vi "filename-manage.vi"(6 "filename pattern":T2, 7 "filename-action":T1=enum."parse", 9 "folder":path=path "C:/data/Ultrasound/birdcage/Hg1201/Test", 11 "file name":string="f027_lsco2_122317.dat") -> (3 "filename OUT":string)   [LabVIEW 2018]
uses:
  filename-pattern.ctl
  filename-action.ctl
  <vilib>/Utility/libraryn.llb/Check if File or Folder Exists.vi
  <vilib>/regexp/Match Regular Expression.xnode
panel:
  out "unique index out":i32
  out "pattern 2":string="^(\\s+)(\\d+)_(.*)_(\\d\\d\\d\\d\\d\\d)\\.dat$"
  out "pattern":string="^(\\s+)(\\d+)_(.*)_(\\d\\d\\d\\d\\d\\d)\\.dat$"
  out "whole match":string
  out "offset past match":i32=-1
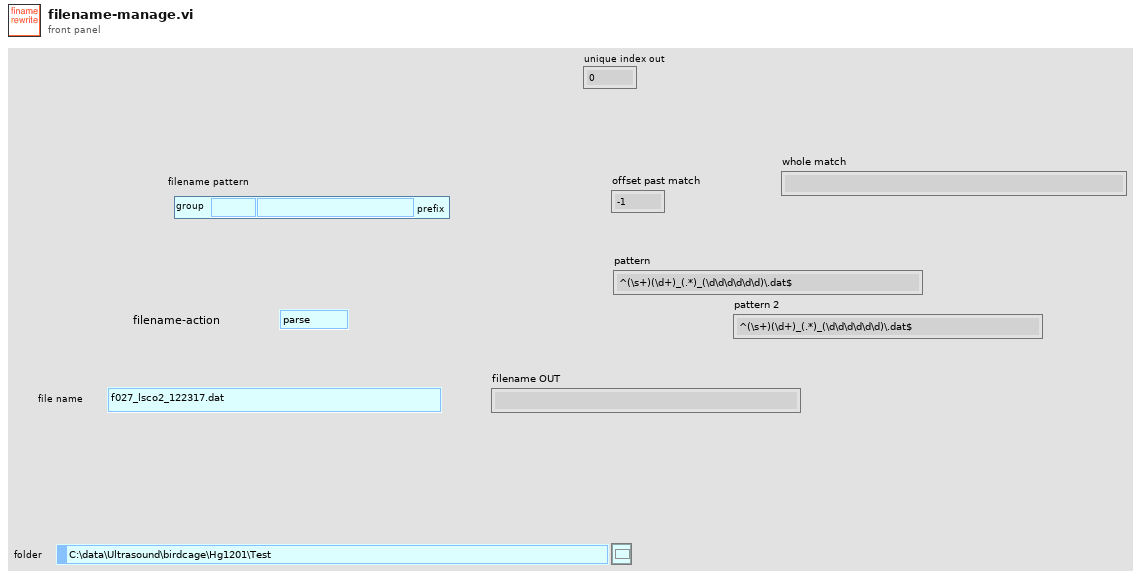
[diagram p1: front panel]
types:
  T1 = typedef "filename-action.ctl" = enum16{"rewrite", "parse", "force pattern", "uniquenum"}
  T2 = typedef "filename-pattern.ctl" = cluster{"prefix":string, "group":string}
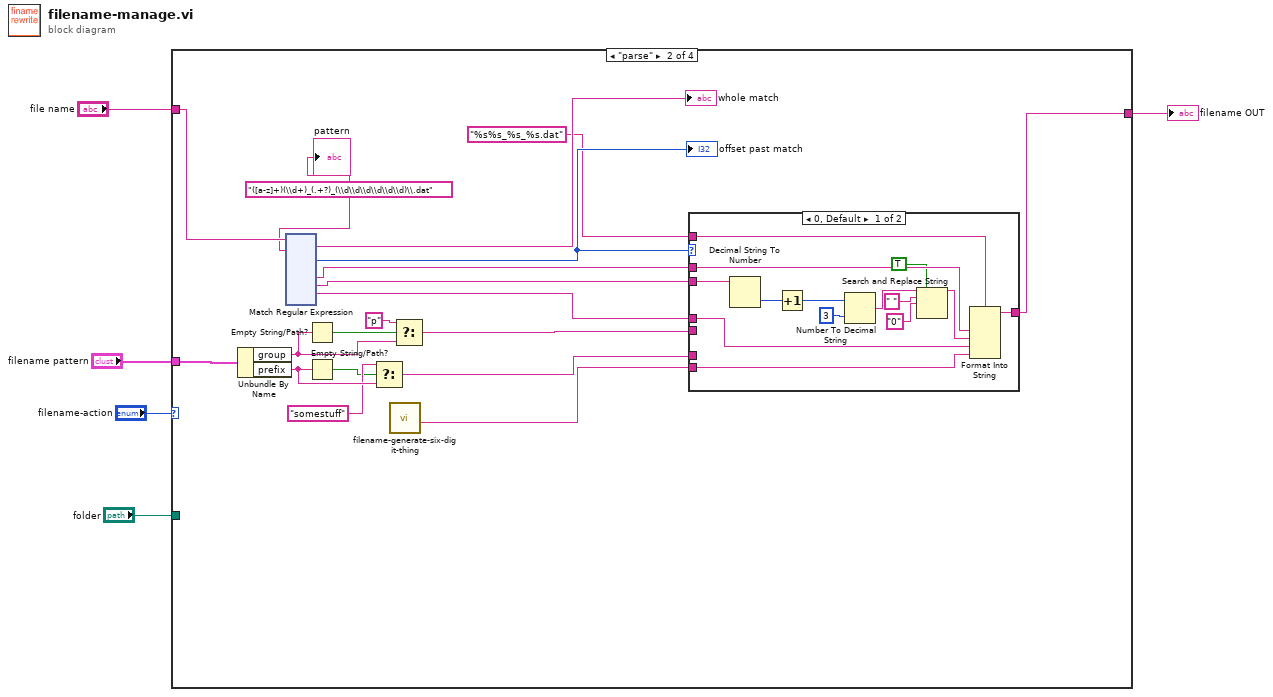
[diagram p0: block diagram]
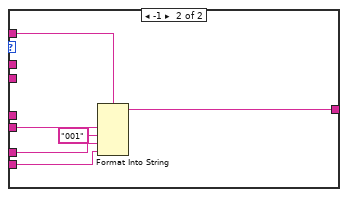
[diagram p3: hidden frame]
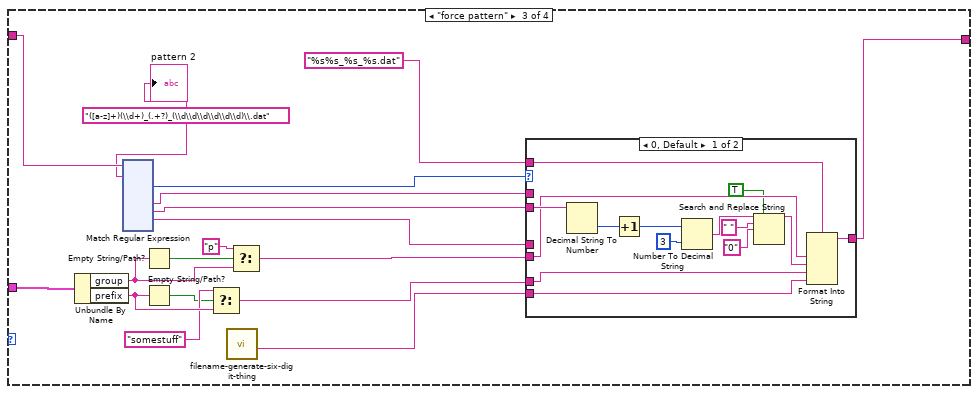
[diagram p4: hidden frame]
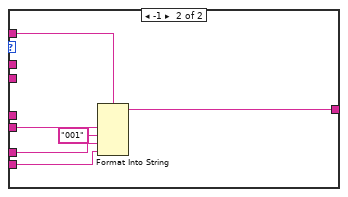
[diagram p5: hidden frame]
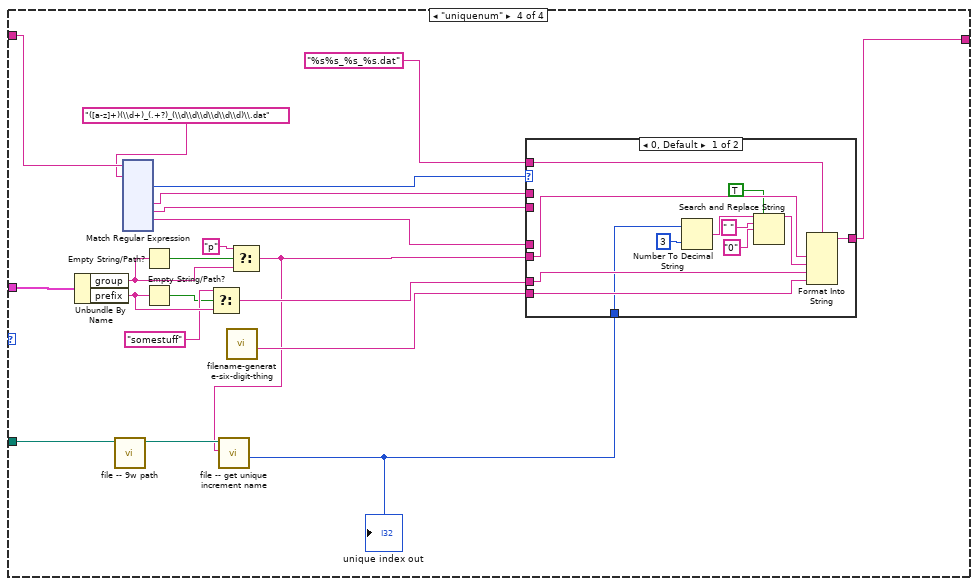
[diagram p6: hidden frame]
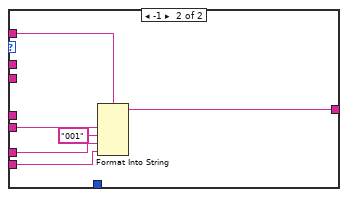
[diagram p7: hidden frame]
diagram:
  n1 = case shown="\"parse\"" "filename-action" {
    tunnel: "file name" -> [w6 w25 w182 w342]
    tunnel: "filename pattern" -> [_ w24 w181 w341]
    tunnel: [w6 w11 w169 w330] -> w2
    tunnel: "folder" -> [_ _ _ w325]
    frame "rewrite", Default {
    }
    frame "parse" {
      w22 = "([a-z]+)(\\d+)_(.+?)_(\\d\\d\\d\\d\\d\\d)\\.dat" ("format string")
      n2 = Unbundle By Name(w24) -> ("group"=w19:string, "prefix"=w18:string)
      n3 = xnode "Match Regular Expression"("input string"=w25, "regular expression"=w22) -> ("whole match"=→"whole match":string, "offset past match"=w15:i32, "submatch 1"=w9:string, "submatch 2"=w8:string, "submatch 3"=w7:string)  [unwired: 4 in, 4 out]
      "offset past match" <- w15
      n4 = Empty String/Path?(string/path=w19) -> (empty?=w21:bool)
      n5 = Empty String/Path?(string/path=w18) -> (empty?=w16:bool)
      n6 = Select(t="somestuff", s=w16, f=w18) -> (s? t:f=w12:string)
      n7 = call "filename-generate-six-digit-thing.vi"() -> ("sixdigit"=w10:string)  [unwired: 9 in, 2 out]
      n8 = Select(t="p", s=w21, f=w19) -> (s? t:f=w13:string)
      n9 = case shown="0, Default" w15 {
        tunnel: "%s%s_%s_%s.dat" ("format string") -> [w28 w45]
        tunnel: w13 -> [_ w44]
        tunnel: w12 -> [_ w43]
        tunnel: [w38 w42] -> w11
        tunnel: w10 -> [w39 w41]
        tunnel: w9 -> [w37 _]
        tunnel: w8 -> [w36 _]
        tunnel: w7 -> [w27 _]
        frame 0, Default {
          n10 = Decimal String To Number(string=w36) -> (number=w35:i32)  [unwired: 2 in, 1 out]
          n11 = Increment(x=w35) -> (x+1=w34:i32)
          n12 = Number To Decimal String(number=w34, width (-)=i16 3) -> (decimal integer string=w30:string)
          n13 = Search and Replace String(replace all?=TRUE ("replace all? (F)"), input string=w30, search string=" ", replace string="0" ("replace string (\"\")")) -> (result string=w29:string)  [unwired: 4 in, 3 out]
          n14 = Format Into String(format string=w28, w37, w29, w27, w39) -> (resulting string=w38:string)  [unwired: 2 in, 1 out]
        }
        frame -1 {
          n15 = Format Into String(format string=w45, w44, "001" ("input 2"), w43, w41) -> (resulting string=w42:string)  [unwired: 2 in, 1 out]
        }
      }
      "pattern" <- w22
    }
    frame "force pattern" {
      w180 = "([a-z]+)(\\d+)_(.+?)_(\\d\\d\\d\\d\\d\\d)\\.dat" ("format string")
      n16 = Unbundle By Name(w181) -> ("group"=w177:string, "prefix"=w176:string)
      n17 = xnode "Match Regular Expression"("input string"=w182, "regular expression"=w180) -> ("offset past match"=w173:i32, "submatch 1"=w167:string, "submatch 2"=w166:string, "submatch 3"=w165:string)  [unwired: 4 in, 5 out]
      n18 = Empty String/Path?(string/path=w177) -> (empty?=w179:bool)
      n19 = Empty String/Path?(string/path=w176) -> (empty?=w174:bool)
      n20 = Select(t="somestuff", s=w174, f=w176) -> (s? t:f=w170:string)
      n21 = call "filename-generate-six-digit-thing.vi"() -> ("sixdigit"=w168:string)  [unwired: 9 in, 2 out]
      n22 = Select(t="p", s=w179, f=w177) -> (s? t:f=w171:string)
      n23 = case shown="0, Default" w173 {
        tunnel: "%s%s_%s_%s.dat" ("format string") -> [w186 w202]
        tunnel: w171 -> [w185 w201]
        tunnel: w170 -> [w184 w200]
        tunnel: [w195 w199] -> w169
        tunnel: w168 -> [w196 w198]
        tunnel: w167 -> [_ _]
        tunnel: w166 -> [w194 _]
        tunnel: w165 -> [_ _]
        frame 0, Default {
          n24 = Decimal String To Number(string=w194) -> (number=w193:i32)  [unwired: 2 in, 1 out]
          n25 = Increment(x=w193) -> (x+1=w192:i32)
          n26 = Number To Decimal String(number=w192, width (-)=i16 3) -> (decimal integer string=w188:string)
          n27 = Search and Replace String(replace all?=TRUE ("replace all? (F)"), input string=w188, search string=" ", replace string="0" ("replace string (\"\")")) -> (result string=w187:string)  [unwired: 4 in, 3 out]
          n28 = Format Into String(format string=w186, w185, w187, w184, w196) -> (resulting string=w195:string)  [unwired: 2 in, 1 out]
        }
        frame -1 {
          n29 = Format Into String(format string=w202, w201, "001" ("input 2"), w200, w198) -> (resulting string=w199:string)  [unwired: 2 in, 1 out]
        }
      }
      "pattern 2" <- w180
    }
    frame "uniquenum" {
      n30 = Unbundle By Name(w341) -> ("group"=w337:string, "prefix"=w336:string)
      n31 = call "file -- 9w path.vi"("sweep folder"=w325) -> ("9w path"=w324:path)  [unwired: 10 in]
      n32 = xnode "Match Regular Expression"("input string"=w342, "regular expression"="([a-z]+)(\\d+)_(.+?)_(\\d\\d\\d\\d\\d\\d)\\.dat" ("format string")) -> ("offset past match"=w333:i32, "submatch 1"=w328:string, "submatch 2"=w327:string, "submatch 3"=w326:string)  [unwired: 4 in, 5 out]
      n33 = Empty String/Path?(string/path=w337) -> (empty?=w339:bool)
      n34 = Empty String/Path?(string/path=w336) -> (empty?=w334:bool)
      n35 = Select(t="somestuff", s=w334, f=w336) -> (s? t:f=w331:string)
      n36 = call "filename-generate-six-digit-thing.vi"() -> ("sixdigit"=w329:string)  [unwired: 9 in, 2 out]
      n37 = Select(t="p", s=w339, f=w337) -> (s? t:f=w323:string)
      n38 = call "file -- get unique increment name.vi"("prefix"=w323, "9w folder path"=w324) -> ("unique index out"=w322:i32)  [unwired: 9 in]
      "unique index out" <- w322
      n39 = case shown="0, Default" w333 {
        tunnel: "%s%s_%s_%s.dat" ("format string") -> [w347 w360]
        tunnel: w323 -> [w346 w359]
        tunnel: w331 -> [w345 w358]
        tunnel: [w353 w357] -> w330
        tunnel: w329 -> [w354 w356]
        tunnel: w328 -> [_ _]
        tunnel: w327 -> [_ _]
        tunnel: w326 -> [_ _]
        tunnel: w322 -> [w344 _]
        frame 0, Default {
          n40 = Number To Decimal String(number=w344, width (-)=i16 3) -> (decimal integer string=w349:string)
          n41 = Search and Replace String(replace all?=TRUE ("replace all? (F)"), input string=w349, search string=" ", replace string="0" ("replace string (\"\")")) -> (result string=w348:string)  [unwired: 4 in, 3 out]
          n42 = Format Into String(format string=w347, w346, w348, w345, w354) -> (resulting string=w353:string)  [unwired: 2 in, 1 out]
        }
        frame -1 {
          n43 = Format Into String(format string=w360, w359, "001" ("input 2"), w358, w356) -> (resulting string=w357:string)  [unwired: 2 in, 1 out]
        }
      }
    }
  }
  "filename OUT" <- w2
